vi "Inversor setup.vi"(8 "error in (no error)":errorcluster) -> (0 "error out":errorcluster, 3 "Module ID":i32)   [LabVIEW 2019]
doc: "_____\nCreated using DQMH Framework: Event Scripter 7.1.0.1503."
uses:
  Libraries/Inversor/Inversor.lvlib
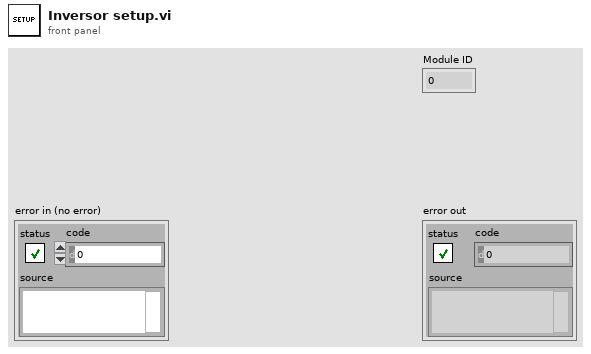
[diagram p1: front panel]
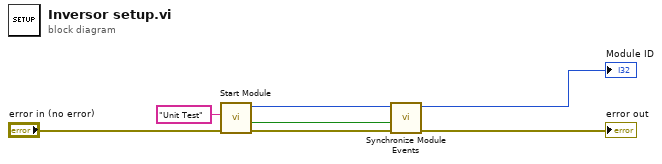
[diagram p0: block diagram]
diagram:
  n1 = call "Start Module.vi"("error in"="error in (no error)", "Nombre"="Unit Test") -> ("error out"=w6:errorcluster, "Wait for Event Sync?"=w2:bool, "Module ID"=w3:i32)  [unwired: 5 in, 2 out]
  n2 = call "Synchronize Module Events.vi"("error in"=w6, "Wait for Event Sync?"=w2, "Module ID in"=w3) -> ("error out"=→"error out":errorcluster, "Module ID out"=→"Module ID":i32)  [unwired: 7 in]
